vi "Facade.vi"(0 "Data In":T6=25.0 min=0.0 max=100.0 step=1.0 scale=0.0..100.0 scale format="%#.1f", 2 "Display State In":T2={"Y_State"={"connect"=FALSE, "Y_State"=enum."initialize", "Y"=0.0}, "Write"=FALSE, "button state"=enum."init", "reset_timer"=FALSE, "load_timer"=FALSE, "end_timer"=TRUE}, 3 "Container State":T5) -> (6 "Data Out":T6=25.0 min=0.0 max=100.0 step=1.0 scale=0.0..100.0 scale format="%#.1f", 7 "Display State Out":T2={"Y_State"={"connect"=FALSE, "Y_State"=enum."initialize", "Y"=0.0}, "Write"=FALSE, "button state"=enum."init", "reset_timer"=FALSE, "load_timer"=FALSE, "end_timer"=TRUE}, 8 "Action":T1)   [LabVIEW 2019, in "Heating.lvlib" / "YQ.xctl"]
uses:
  YQ.xctl
  Data.ctl
  <vilib>/_xctls/Container State.ctl
  State.ctl
  Y_state.ctl
  Y_controlState.ctl
  <vilib>/_xctls/Action.ctl
  <vilib>/_xctls/XControlSupport.lvlib
  Timer Delay/Timers.lvlib
  Heating.lvlib
panel:
  in  "manual control":dbl(slide)=25.0 caption="%" min=0.0 max=100.0 step=1.0 scale=0.0..100.0 scale format="%#.1f"
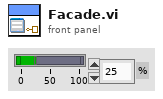
[diagram p1: front panel]
types:
  T1 = typedef "XControlSupport.lvlib/Action.ctl" = cluster{"Data Changed?":bool, "State Changed?":bool, "Action Name":string}
  T2 = typedef "Heating.lvlib/YQ.xctl/State.ctl" = cluster{"Y_State":cluster{"connect":bool, "Y_State":T3, "Y":dbl}, "Write":bool, "button state":T4, "reset_timer":bool, "load_timer":bool, "end_timer":bool}
  T3 = typedef "Heating.lvlib/Y_state.ctl" = enum8{"initialize", "alarm", "min", "stop", "hand", "auto", "max"}
  T4 = typedef "Heating.lvlib/YQ.xctl/Y_controlState.ctl" = enum16{"init", "not connect", "alarm", "min", "stop", "hand", "value change", "auto", "max"}
  T5 = typedef "XControlSupport.lvlib/Container State.ctl" = cluster{"Indicator?":bool, "Run Mode?":bool, " Refnum":refnum<vi>}
  T6 = typedef "Heating.lvlib/YQ.xctl/Data.ctl" = dbl
  T7 = enum8{"Enabled", "Disabled", "Disabled and Grayed Out"}
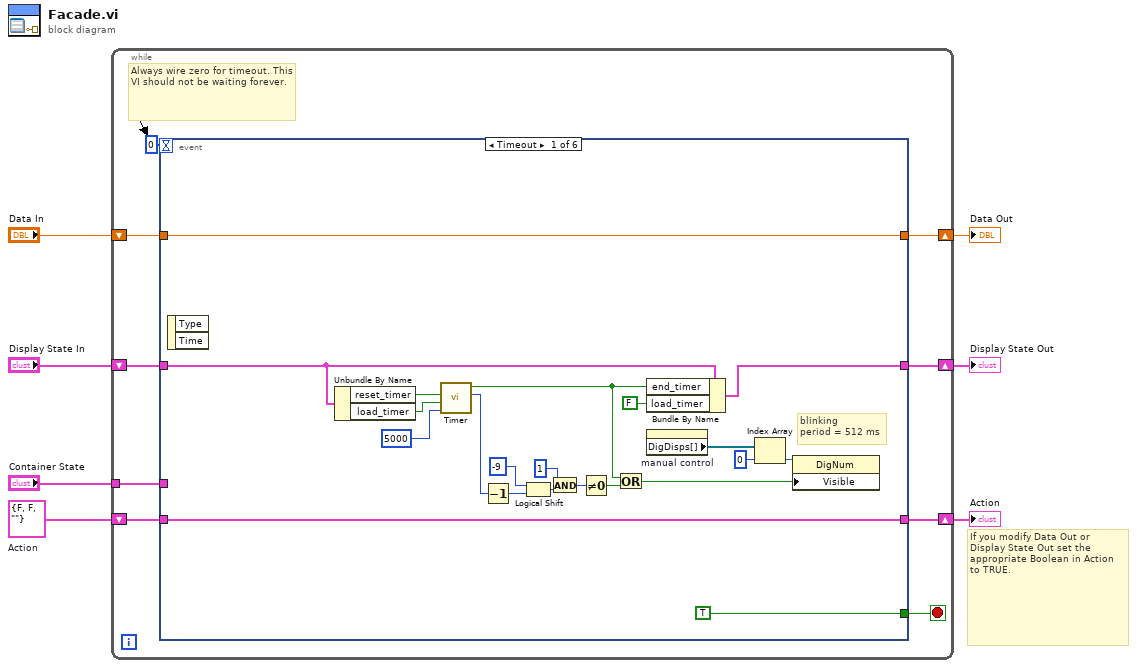
[diagram p0: block diagram]
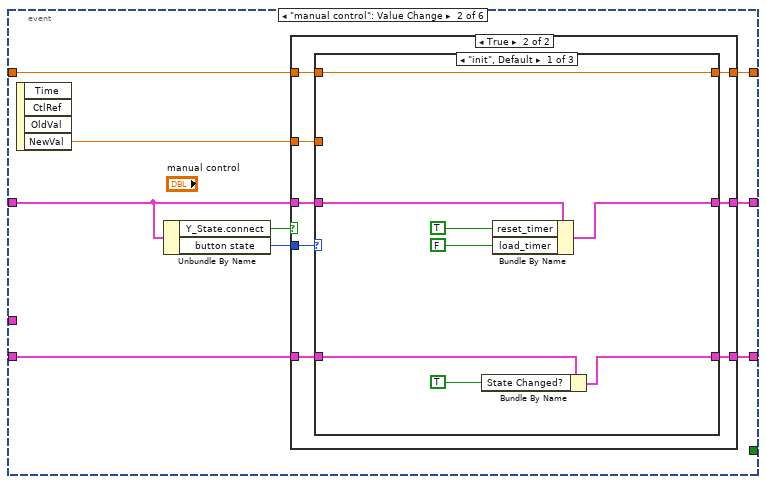
[diagram p2: hidden frame]
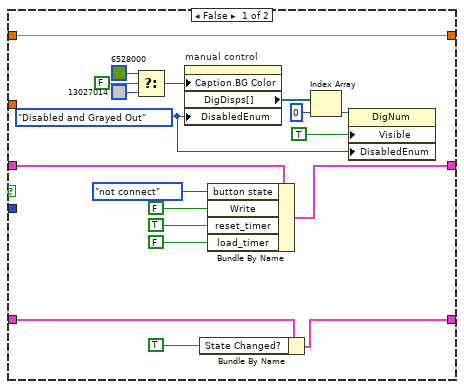
[diagram p3: hidden frame]
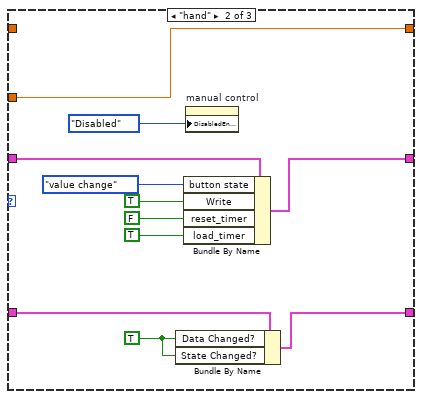
[diagram p4: hidden frame]
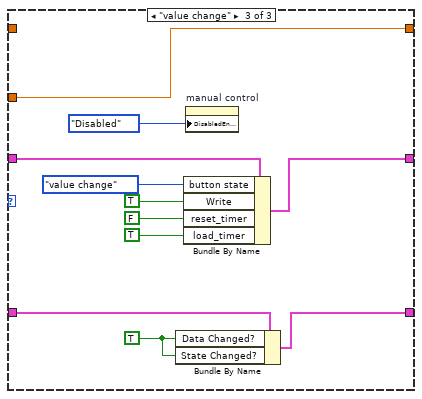
[diagram p5: hidden frame]
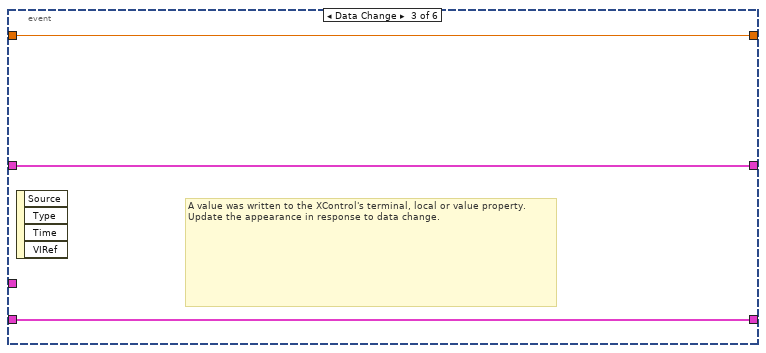
[diagram p6: hidden frame]
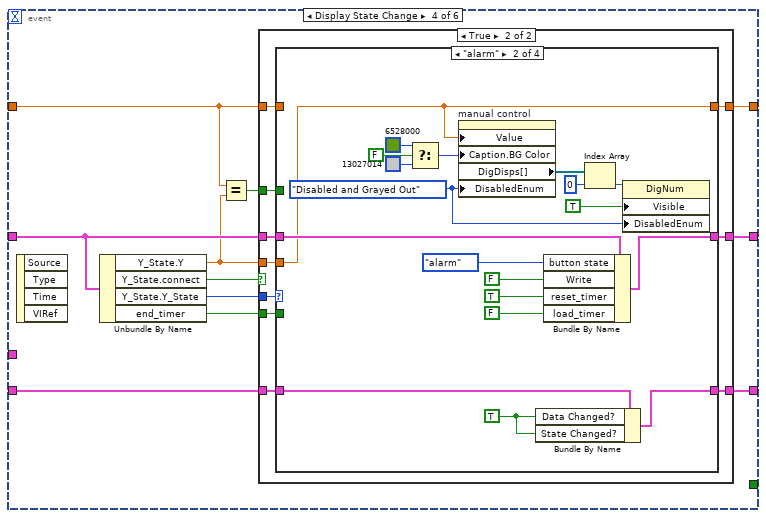
[diagram p7: hidden frame]
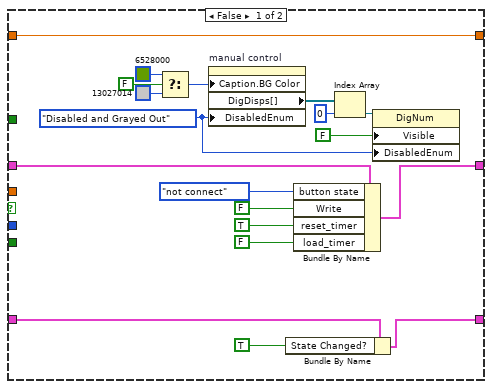
[diagram p8: hidden frame]
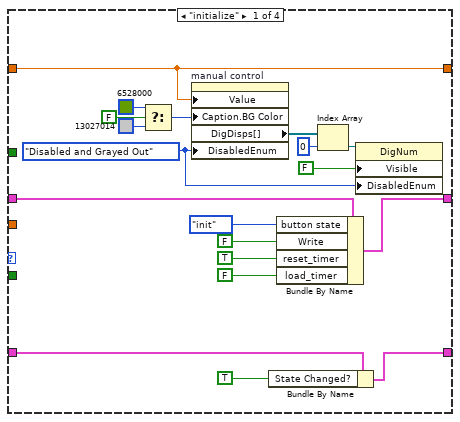
[diagram p9: hidden frame]
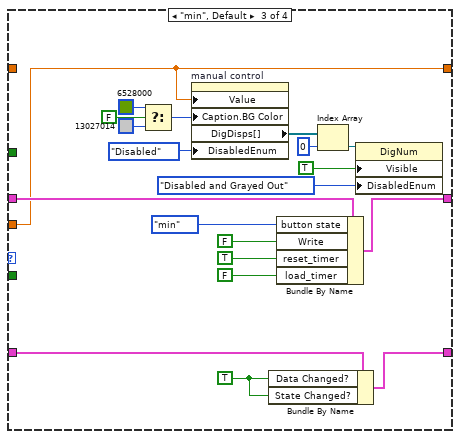
[diagram p10: hidden frame]
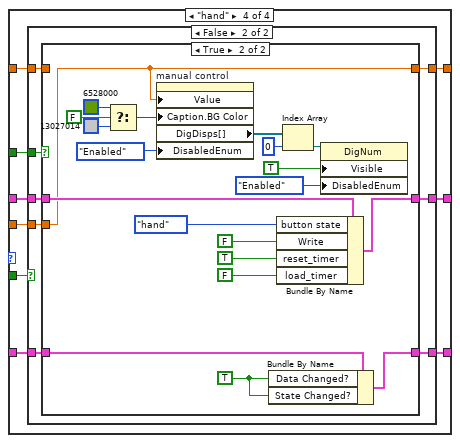
[diagram p11: hidden frame]
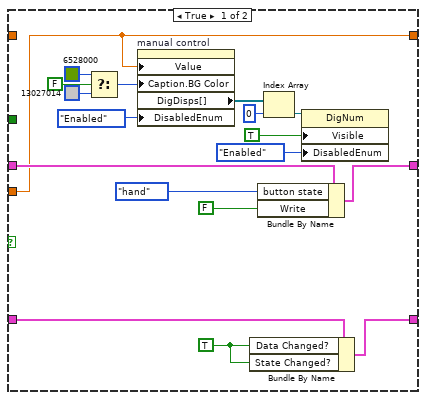
[diagram p12: hidden frame]
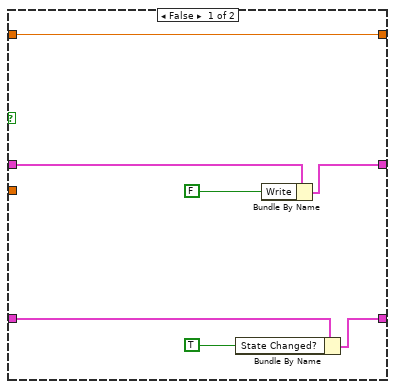
[diagram p13: hidden frame]
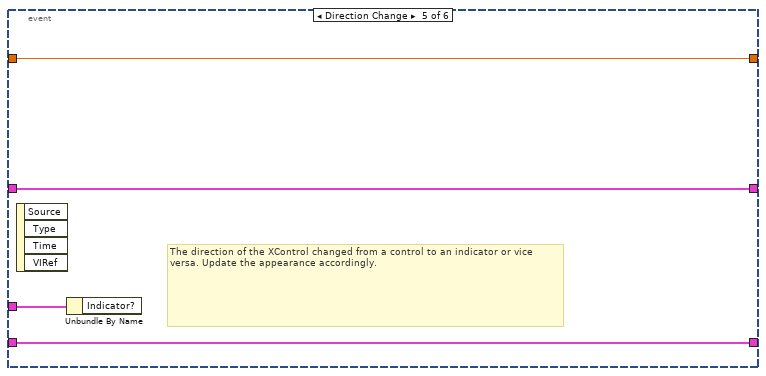
[diagram p14: hidden frame]
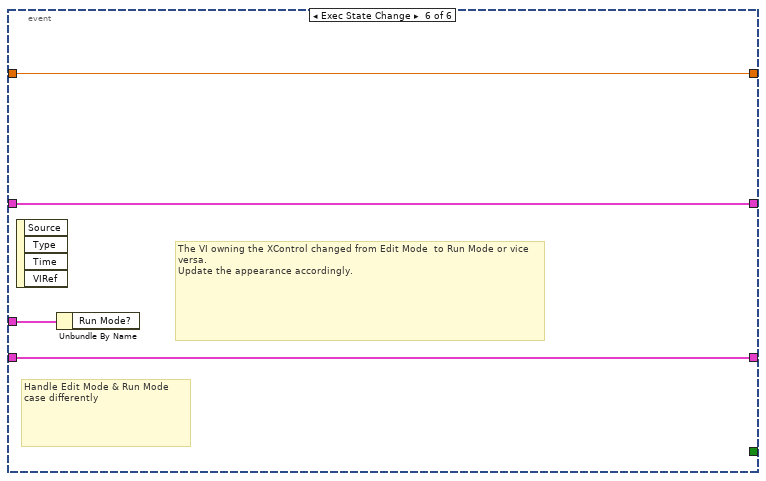
[diagram p15: hidden frame]
diagram:
  w1 = T1 {"Data Changed?"=FALSE, "State Changed?"=FALSE, "Action Name"=""}  # Action
  # "If you modify Data Out or\nDisplay State Out set the\nappropriate Boolean in Action\nto TRUE."
  n1 = while {
    shift-right: [w8] -> w4
    shift-left: "Display State In" -> [w16]
    tunnel: "Container State" -> [w13]
    shift-right: [w11] -> w7
    shift-left: "Data In" -> [w12]
    shift-right: [w9] -> w2
    shift-left: w1 -> [w10]
    stop <- w15 stop-if-true
    # "Always wire zero for timeout. This\nVI should not be waiting forever."
    n2 = event shown="[0] Timeout" {
      selector: _ -> [_ _ _ _ _ _]
      dyn-events: _ -> [_ _ _ _ _ _]
      timeout: 0 -> [_ _ _ _ _ _]
      tunnel: w16 -> [w32 w41 w105 w112 w269 w273]
      tunnel: [w31 w46 w105 w116 w269 w273] -> w8
      tunnel: [TRUE _ _ _ _ _] -> w15
      tunnel: w13 -> [_ _ _ _ w270 w274]
      tunnel: w12 -> [w35 w45 w106 w108 w268 w272]
      tunnel: [w35 w44 w106 w117 w268 w272] -> w11
      tunnel: [w36 w42 w104 w114 w267 w271] -> w9
      tunnel: w10 -> [w36 w43 w104 w115 w267 w271]
      event Timeout {
        # "blinking\nperiod = 512 ms"
        n3 = event-data() -> ()  [unwired: 1 in, 2 out]
        n4 = Unbundle By Name(w32) -> ("reset_timer"=w34:bool, "load_timer"=w33:bool)
        n5 = call "Timer.vi"("ms"=5000, "Load (F)"=w33, "Reset (F)"=w34) -> ("t ms"=w29:u32, "End"=w26:bool)  [unwired: 6 in]
        n6 = Decrement(x=w29) -> (x-1=w25:u32)
        n7 = Logical Shift(y=i16 -9, x=w25) -> (x << y=w23:u32)
        n8 = And(x=u32 1 ("y"), y=w23) -> (x .and. y?=w21:u32)
        n9 = Not Equal To 0?(x=w21) -> (x != 0?=w27:bool)
        n10 = Or(x=w26, y=w27) -> (x .or. y?=w17:bool)
        n11 = Bundle By Name(cluster=w32, "end_timer"=w26, "load_timer"=FALSE) -> (w31:T2)
        n12 = property on="manual control" class="Slide (strict)"() -> ("DigDisps[]"=w19:refnum<vi>[])  [unwired: 2 in, 2 out]
        n13 = Index Array(array=w19, index=0) -> (element=w20:refnum<vi>)
        n14 = property class="DigNum"(reference=w20, "Visible"=w17) -> ()  [unwired: 1 in, 2 out]
      }
      event "manual control": Value Change {
        n15 = event-data() -> ("NewVal"=w38:dbl)  [unwired: 1 in, 3 out]
        n16 = Unbundle By Name(w41) -> ("Y_State.connect"=w40:bool, "button state"=w39:T4)
        n17 = case shown="True" w40 {
          tunnel: w39 -> [_ w73]
          tunnel: w38 -> [_ w72]
          tunnel: w41 -> [w64 w71]
          tunnel: [w63 w70] -> w46
          tunnel: w45 -> [w49 w69]
          tunnel: [w49 w68] -> w44
          tunnel: w43 -> [w61 w66]
          tunnel: [w60 w67] -> w42
          frame False {
            w47 = T7."Disabled and Grayed Out" ("Disabled")
            n18 = Select(t=u32 6528000, s=FALSE, f=u32 13027014) -> (s? t:f=w48:u32)
            n19 = property on="manual control" class="Slide (strict)"("Caption.BG Color"=w48, "DisabledEnum"=w47) -> ("DigDisps[]"=w55:refnum<vi>[])  [unwired: 2 in, 2 out]
            n20 = Bundle By Name(cluster=w61, "State Changed?"=TRUE ("Data Changed?")) -> (w60:T1)
            n21 = Bundle By Name(cluster=w64, "button state"=Y_controlState."not connect" ("f 3"), "Write"=FALSE ("Z_ASwitch"), "reset_timer"=TRUE ("Z_ASwitch"), "load_timer"=FALSE ("Z_ASwitch")) -> (w63:T2)
            n22 = Index Array(array=w55, index=0) -> (element=w56:refnum<vi>)
            n23 = property class="DigNum"(reference=w56, "Visible"=TRUE ("Z_ASwitch"), "DisabledEnum"=w47) -> ()  [unwired: 1 in, 2 out]
          }
          frame True {
            n24 = case shown="\"init\", Default" w73 {
              tunnel: w72 -> [_ w90 w101]
              tunnel: w71 -> [w80 w92 w103]
              tunnel: [w79 w91 w102] -> w70
              tunnel: w69 -> [w78 _ _]
              tunnel: [w78 w90 w101] -> w68
              tunnel: [w75 w88 w99] -> w67
              tunnel: w66 -> [w76 w89 w100]
              frame "init", Default {
                # "local hand"
                n25 = Bundle By Name(cluster=w76, "State Changed?"=TRUE ("Data Changed?")) -> (w75:T1)
                n26 = Bundle By Name(cluster=w80, "reset_timer"=TRUE, "load_timer"=FALSE) -> (w79:T2)
              }
              frame "hand" {
                w83 = TRUE ("Data Changed?")
                # "local hand"
                n27 = Bundle By Name(cluster=w89, "Data Changed?"=w83, "State Changed?"=w83) -> (w88:T1)
                n28 = Bundle By Name(cluster=w92, "button state"=Y_controlState."value change" ("f 3"), "Write"=TRUE ("Z_ASwitch"), "reset_timer"=FALSE ("Z_ASwitch"), "load_timer"=TRUE ("Z_ASwitch")) -> (w91:T2)
                n29 = property on="manual control" class="Slide (strict)"("DisabledEnum"=T7."Disabled" ("Disabled")) -> ()  [unwired: 2 in, 2 out]
              }
              frame "value change" {
                w94 = TRUE ("Data Changed?")
                # "local hand"
                n30 = Bundle By Name(cluster=w100, "Data Changed?"=w94, "State Changed?"=w94) -> (w99:T1)
                n31 = Bundle By Name(cluster=w103, "button state"=Y_controlState."value change" ("f 3"), "Write"=TRUE ("Z_ASwitch"), "reset_timer"=FALSE ("Z_ASwitch"), "load_timer"=TRUE ("Z_ASwitch")) -> (w102:T2)
                n32 = property on="manual control" class="Slide (strict)"("DisabledEnum"=T7."Disabled" ("Disabled")) -> ()  [unwired: 2 in, 2 out]
              }
            }
          }
        }
      }
      event Data Change {
        # "A value was written to the XControl's terminal, local or value property.\nUpdate the appearance in response to data change."
        n33 = event-data() -> ()  [unwired: 1 in, 4 out]
      }
      event Display State Change {
        n34 = event-data() -> ()  [unwired: 1 in, 4 out]
        n35 = Unbundle By Name(w112) -> ("Y_State.Y"=w109:dbl, "Y_State.connect"=w113:bool, "Y_State.Y_State"=w110:T3, "end_timer"=w111:bool)
        n36 = Equal?(x=w108, y=w109) -> (x = y?=w107:bool)
        n37 = case shown="True" w113 {
          tunnel: w110 -> [_ w146]
          tunnel: w112 -> [w135 w145]
          tunnel: [w134 w144] -> w116
          tunnel: w108 -> [w119 w143]
          tunnel: [w119 w142] -> w117
          tunnel: w115 -> [w132 w140]
          tunnel: [w131 w141] -> w114
          tunnel: w111 -> [_ w139]
          tunnel: w109 -> [_ w138]
          tunnel: w107 -> [_ w137]
          frame False {
            w118 = T7."Disabled and Grayed Out" ("Disabled")
            n38 = Select(t=u32 6528000, s=FALSE, f=u32 13027014) -> (s? t:f=w120:u32)
            n39 = property on="manual control" class="Slide (strict)"("Caption.BG Color"=w120, "DisabledEnum"=w118) -> ("DigDisps[]"=w126:refnum<vi>[])  [unwired: 2 in, 2 out]
            n40 = Bundle By Name(cluster=w132, "State Changed?"=TRUE ("Data Changed?")) -> (w131:T1)
            n41 = Bundle By Name(cluster=w135, "button state"=Y_controlState."not connect" ("f 3"), "Write"=FALSE ("Z_ASwitch"), "reset_timer"=TRUE ("Z_ASwitch"), "load_timer"=FALSE ("Z_ASwitch")) -> (w134:T2)
            n42 = Index Array(array=w126, index=0) -> (element=w127:refnum<vi>)
            n43 = property class="DigNum"(reference=w127, "Visible"=FALSE ("Z_ASwitch"), "DisabledEnum"=w118) -> ()  [unwired: 1 in, 2 out]
          }
          frame True {
            n44 = case shown="\"alarm\"" w146 {
              tunnel: w145 -> [w165 w184 w204 w213]
              tunnel: [w164 w183 w203 w212] -> w144
              tunnel: w143 -> [w147 _ _ w206]
              tunnel: [w147 w166 w185 w207] -> w142
              tunnel: [w162 w181 w201 w210] -> w141
              tunnel: w140 -> [w163 w182 w202 w211]
              tunnel: w139 -> [_ _ _ w209]
              tunnel: w138 -> [_ w166 w185 w208]
              tunnel: w137 -> [_ _ _ w205]
              frame "initialize" {
                w156 = T7."Disabled and Grayed Out" ("Disabled")
                # "local hand"
                n45 = Select(t=u32 6528000, s=FALSE, f=u32 13027014) -> (s? t:f=w148:u32)
                n46 = property on="manual control" class="Slide (strict)"("Value"=w147, "Caption.BG Color"=w148, "DisabledEnum"=w156) -> ("DigDisps[]"=w154:refnum<vi>[])  [unwired: 2 in, 2 out]
                n47 = Bundle By Name(cluster=w163, "State Changed?"=TRUE ("Data Changed?")) -> (w162:T1)
                n48 = Bundle By Name(cluster=w165, "button state"=Y_controlState."init" ("f 3"), "Write"=FALSE ("Z_ASwitch"), "reset_timer"=TRUE ("Z_ASwitch"), "load_timer"=FALSE ("Z_ASwitch")) -> (w164:T2)
                n49 = Index Array(array=w154, index=0) -> (element=w155:refnum<vi>)
                n50 = property class="DigNum"(reference=w155, "Visible"=FALSE ("Z_ASwitch"), "DisabledEnum"=w156) -> ()  [unwired: 1 in, 2 out]
              }
              frame "alarm" {
                w175 = T7."Disabled and Grayed Out" ("Disabled")
                w176 = TRUE ("Data Changed?")
                # "local hand"
                n51 = Select(t=u32 6528000, s=FALSE, f=u32 13027014) -> (s? t:f=w167:u32)
                n52 = property on="manual control" class="Slide (strict)"("Value"=w166, "Caption.BG Color"=w167, "DisabledEnum"=w175) -> ("DigDisps[]"=w173:refnum<vi>[])  [unwired: 2 in, 2 out]
                n53 = Bundle By Name(cluster=w182, "Data Changed?"=w176, "State Changed?"=w176) -> (w181:T1)
                n54 = Bundle By Name(cluster=w184, "button state"=Y_controlState."alarm" ("f 3"), "Write"=FALSE ("Z_ASwitch"), "reset_timer"=TRUE ("Z_ASwitch"), "load_timer"=FALSE ("Z_ASwitch")) -> (w183:T2)
                n55 = Index Array(array=w173, index=0) -> (element=w174:refnum<vi>)
                n56 = property class="DigNum"(reference=w174, "Visible"=TRUE ("Z_ASwitch"), "DisabledEnum"=w175) -> ()  [unwired: 1 in, 2 out]
              }
              frame "min", Default {
                w196 = TRUE ("Data Changed?")
                # "local hand"
                n57 = Select(t=u32 6528000, s=FALSE, f=u32 13027014) -> (s? t:f=w187:u32)
                n58 = property on="manual control" class="Slide (strict)"("Value"=w185, "Caption.BG Color"=w187, "DisabledEnum"=T7."Disabled" ("Disabled")) -> ("DigDisps[]"=w193:refnum<vi>[])  [unwired: 2 in, 2 out]
                n59 = Bundle By Name(cluster=w202, "Data Changed?"=w196, "State Changed?"=w196) -> (w201:T1)
                n60 = Bundle By Name(cluster=w204, "button state"=Y_controlState."min" ("f 3"), "Write"=FALSE ("Z_ASwitch"), "reset_timer"=TRUE ("Z_ASwitch"), "load_timer"=FALSE ("Z_ASwitch")) -> (w203:T2)
                n61 = Index Array(array=w193, index=0) -> (element=w194:refnum<vi>)
                n62 = property class="DigNum"(reference=w194, "Visible"=TRUE ("Z_ASwitch"), "DisabledEnum"=T7."Disabled and Grayed Out" ("Disabled")) -> ()  [unwired: 1 in, 2 out]
              }
              frame "hand" {
                # "local hand"
                n63 = case shown="False" w209 {
                  tunnel: w213 -> [w231 w239]
                  tunnel: [w230 w238] -> w212
                  tunnel: w211 -> [w229 w237]
                  tunnel: [w228 w236] -> w210
                  tunnel: w208 -> [w214 w233]
                  tunnel: [w214 w235] -> w207
                  tunnel: w206 -> [_ w234]
                  tunnel: w205 -> [_ w232]
                  frame True {
                    w225 = TRUE ("Data Changed?")
                    n64 = Select(t=u32 6528000, s=FALSE, f=u32 13027014) -> (s? t:f=w216:u32)
                    n65 = property on="manual control" class="Slide (strict)"("Value"=w214, "Caption.BG Color"=w216, "DisabledEnum"=T7."Enabled" ("Disabled")) -> ("DigDisps[]"=w222:refnum<vi>[])  [unwired: 2 in, 2 out]
                    n66 = Bundle By Name(cluster=w229, "Data Changed?"=w225, "State Changed?"=w225) -> (w228:T1)
                    n67 = Bundle By Name(cluster=w231, "button state"=Y_controlState."hand" ("f 3"), "Write"=FALSE ("Z_ASwitch")) -> (w230:T2)
                    n68 = Index Array(array=w222, index=0) -> (element=w223:refnum<vi>)
                    n69 = property class="DigNum"(reference=w223, "Visible"=TRUE ("Z_ASwitch"), "DisabledEnum"=T7."Enabled" ("Disabled")) -> ()  [unwired: 1 in, 2 out]
                  }
                  frame False {
                    n70 = case shown="True" w232 {
                      tunnel: w239 -> [w242 w266]
                      tunnel: [w241 w265] -> w238
                      tunnel: w237 -> [w245 w264]
                      tunnel: [w243 w263] -> w236
                      tunnel: [w246 w247] -> w235
                      tunnel: w234 -> [w246 _]
                      tunnel: w233 -> [_ w247]
                      frame False {
                        n71 = Bundle By Name(cluster=w245, "State Changed?"=TRUE ("Data Changed?")) -> (w243:T1)
                        n72 = Bundle By Name(cluster=w242, "Write"=FALSE ("Z_ASwitch")) -> (w241:T2)
                      }
                      frame True {
                        w260 = TRUE ("Data Changed?")
                        n73 = Select(t=u32 6528000, s=FALSE, f=u32 13027014) -> (s? t:f=w251:u32)
                        n74 = property on="manual control" class="Slide (strict)"("Value"=w247, "Caption.BG Color"=w251, "DisabledEnum"=T7."Enabled" ("Disabled")) -> ("DigDisps[]"=w257:refnum<vi>[])  [unwired: 2 in, 2 out]
                        n75 = Bundle By Name(cluster=w264, "Data Changed?"=w260, "State Changed?"=w260) -> (w263:T1)
                        n76 = Bundle By Name(cluster=w266, "button state"=Y_controlState."hand" ("f 3"), "Write"=FALSE ("Z_ASwitch"), "reset_timer"=TRUE ("Z_ASwitch"), "load_timer"=FALSE ("Z_ASwitch")) -> (w265:T2)
                        n77 = Index Array(array=w257, index=0) -> (element=w258:refnum<vi>)
                        n78 = property class="DigNum"(reference=w258, "Visible"=TRUE ("Z_ASwitch"), "DisabledEnum"=T7."Enabled" ("Disabled")) -> ()  [unwired: 1 in, 2 out]
                      }
                    }
                  }
                }
              }
            }
          }
        }
      }
      event Direction Change {
        # "The direction of the XControl changed from a control to an indicator or vice versa. Update the appearance accordingly."
        n79 = event-data() -> ()  [unwired: 1 in, 4 out]
        n80 = Unbundle By Name(w270) -> ()  [unwired: 1 out]
      }
      event Exec State Change {
        # "The VI owning the XControl changed from Edit Mode  to Run Mode or vice versa.\nUpdate the appearance accordingly."
        # "Handle Edit Mode & Run Mode\ncase differently"
        n81 = event-data() -> ()  [unwired: 1 in, 4 out]
        n82 = Unbundle By Name(w274) -> ()  [unwired: 1 out]
      }
    }
  }
  "Display State Out" <- w4
  "Data Out" <- w7
  "Action" <- w2
